vi "Subset (multiple).vi"(8 "error in (no error)":errorcluster, 9 "Subset Method":enum16{"Slider (%)", "X[] min and max"}(ring)=enum."X[] min and max", 10 "Subset Slider":cluster{dbl, dbl}(slide)={75.0, 25.0} scale=0.0..100.0 scale format="%#_6f", 11 "XY-data":cluster{"X-array":dbl[], "Y-array":dbl[]}[](array[cluster]) {"Y-array" format="%.2p"; "X-array" format="%.2p"}) -> (0 "error out":errorcluster, 3 "Subset XY-data out":cluster{"X-array":dbl[], "Y-array":dbl[]}[](array[cluster]) {"Y-array" format="%.2p"; "X-array" format="%.2p"})   [LabVIEW 2019, in "xy_utilities.lvlib"]
doc: "Returns a subset of <b>XY-data</b>\n\n<b>Subset Method</b>: choose how to define the subset.\n- <b>X[] min and max</b>: returns subset of data between found maximum and minimum values of <b>x-array</b>. Returns data in ascending x order.\n- <b>Slider (%)</b>: chooses data subset based on percentages (%) defined by <b>Subset Slider</b> \n\nWire data to the data input to determine the polymorphic instance to use or manually select the instance."
uses:
  xy_utilities.lvlib
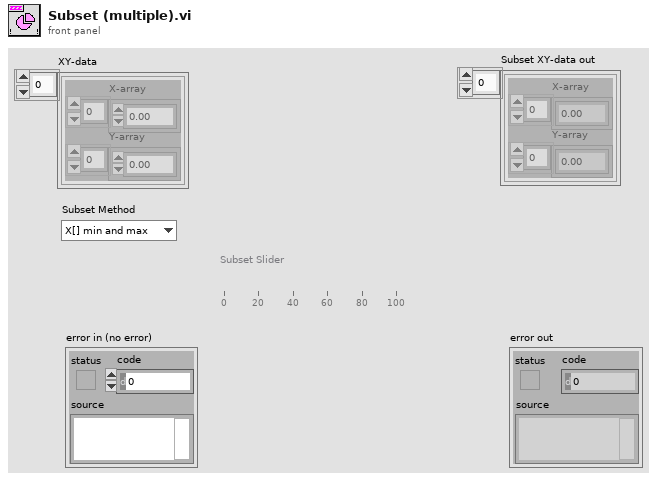
[diagram p1: front panel]
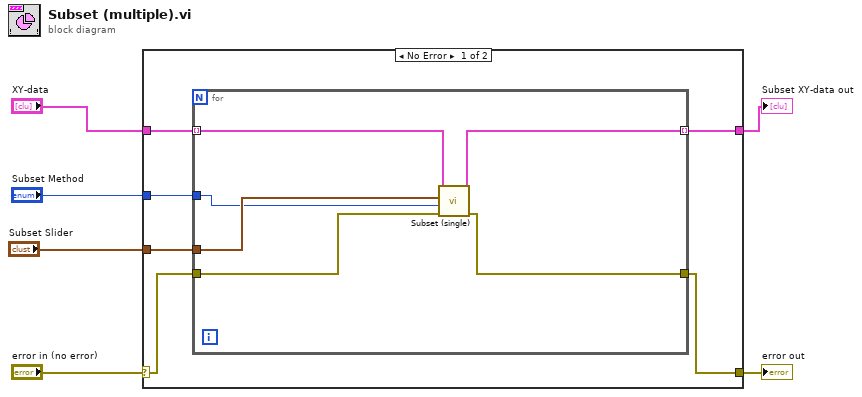
[diagram p0: block diagram]
diagram:
  n1 = case shown="No Error" "error in (no error)" {
    selector: "error in (no error)" -> [w8 w20]
    tunnel: [w7 w20] -> w5
    tunnel: "XY-data" -> [w12 w19]
    tunnel: [w9 w19] -> w3
    tunnel: "Subset Method" -> [w10 _]
    tunnel: "Subset Slider" -> [w11 _]
    frame No Error {
      n2 = for {
        tunnel: w12 -> [w14] mode=indexing
        tunnel: w11 -> [w18]
        tunnel: w10 -> [w17]
        tunnel: [w13] -> w9 mode=indexing
        tunnel: w8 -> [w16]
        tunnel: [w15] -> w7
        n3 = call "Subset (single).vi"("error in (no error)"=w16, "Subset Method"=w17, "Subset Slider (%)"=w18, "XY-data"=w14) -> ("error out"=w15:errorcluster, "XY-data out"=w13:cluster{"X-array":dbl[], "Y-array":dbl[]})  [unwired: 6 in]
      }
    }
    frame Error {
    }
  }
  "error out" <- w5
  "Subset XY-data out" <- w3
